vi "Get Selected Type.vi"(0 "Select Type":T1, 11 "error in (no error)":errorcluster) -> (4 "Selected File Types[]":string[](array[string]), 15 "error out":errorcluster)   [LabVIEW 2016, in "SLL Add Copyright.lvlib"]
uses:
  SLL Add Copyright.lvlib
  _Typedefs/Select File Type.ctl
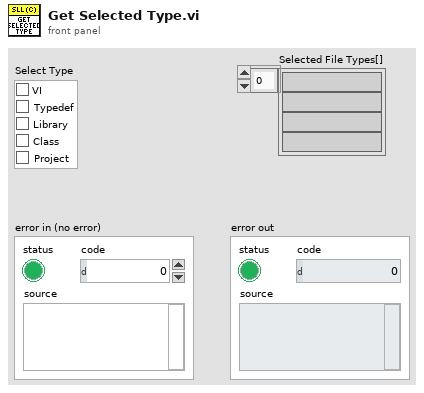
[diagram p1: front panel]
types:
  T1 = typedef "SLL Add Copyright.lvlib/Select File Type.ctl" = cluster{"vi":bool, "ctl":bool, "lvlib":bool, "lvclass":bool, "lvproj":bool}
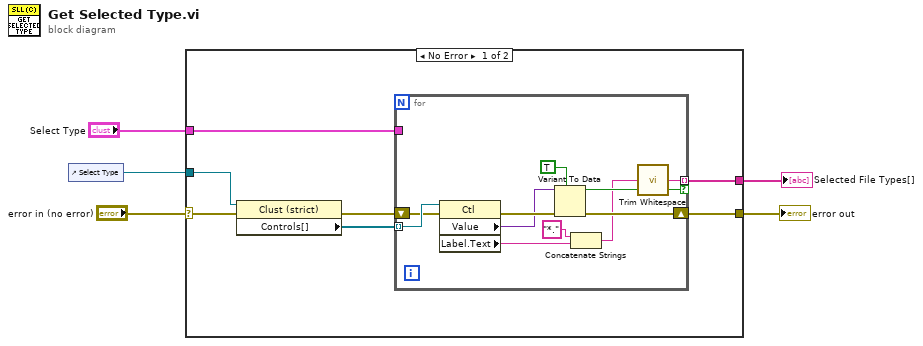
[diagram p0: block diagram]
diagram:
  n1 = control-ref of="Select Type"() -> (w3:refnum<vi>)
  n2 = case shown="No Error" "error in (no error)" {
    selector: "error in (no error)" -> [w10 w24]
    tunnel: [w9 w24] -> w4
    tunnel: w3 -> [w8 _]
    tunnel: [w7 _] -> w2
    tunnel: "Select Type" -> [w6 _]
    frame No Error {
      n3 = property class="Clust (strict)"(reference=w8, error in=w10) -> (error out=w11:errorcluster, "Controls[]"=w12:refnum<vi>[])  [unwired: 1 out]
      n4 = for {
        tunnel: w12 -> [w23] mode=indexing
        tunnel: [w16] -> w7 mode=indexing if=w20
        shift-right: [w18] -> w9
        shift-left: w11 -> [w19]
        tunnel: w6 -> [_]
        n5 = property class="Ctl"(reference=w23, error in=w19) -> (error out=w22:errorcluster, "Value"=w17:variant, "Label.Text"=w14:string)  [unwired: 1 out]
        n6 = Variant To Data(error in=w22, type=TRUE, Variant=w17) -> (data=w20:bool, error out=w18:errorcluster)
        n7 = Concatenate Strings("*." ("string"), w14) -> (w13:string)
        n8 = call <vilib>:"Trim Whitespace.vi"("string"=w13) -> ("trimmed string"=w16:string)  [unwired: 1 in]
      }
    }
    frame Error {
    }
  }
  "error out" <- w4
  "Selected File Types[]" <- w2
